vi "Lab Panel V4.83.vi"() -> ()   [LabVIEW 2013] (continued)
                n1629 = property on="O/I  LAB04-2" class="Bool (strict)"("DisabledEnum"=w2561) -> ()  [unwired: 2 in, 2 out]
                n1630 = property on="O/I  LAB03-2" class="Bool (strict)"("DisabledEnum"=w2563) -> ()  [unwired: 2 in, 2 out]
                n1631 = Not(x=w2568) -> (.not. x?=w2569:bool)
                n1632 = Not(x=w2567) -> (.not. x?=w2570:bool)
                n1633 = Not(x=w2566) -> (.not. x?=w2571:bool)
                n1634 = property on="RESULT LAB05-2" class="Bool (strict)"("Visible"=w2569) -> ()  [unwired: 2 in, 2 out]
                n1635 = property on="RESULT LAB05-1" class="Bool (strict)"("Visible"=w2570) -> ()  [unwired: 2 in, 2 out]
                n1636 = Not(x=w2565) -> (.not. x?=w2572:bool)
                n1637 = property on="RESULT LAB04-2" class="Bool (strict)"("Visible"=w2571) -> ()  [unwired: 2 in, 2 out]
                n1638 = Not(x=w2564) -> (.not. x?=w2573:bool)
                n1639 = property on="RESULT LAB04-1" class="Bool (strict)"("Visible"=w2572) -> ()  [unwired: 2 in, 2 out]
                n1640 = property on="RESULT LAB03-2" class="Bool (strict)"("Visible"=w2573) -> ()  [unwired: 2 in, 2 out]
              }
              frame #2 {
                # "disable calibrate if any test running"
                n1641 = Or(x=w2595, y=w2594) -> (x .or. y?=w2588:bool)
                n1642 = Or(x=w2597, y=w2596) -> (x .or. y?=w2590:bool)
                n1643 = Or(x=w2601, y=w2600) -> (x .or. y?=w2592:bool)
                n1644 = Or(x=w2599, y=w2598) -> (x .or. y?=w2591:bool)
                n1645 = Or(x=w2603, y=w2602) -> (x .or. y?=w2593:bool)
                n1646 = Or(x=w2591, y=w2590) -> (x .or. y?=w2589:bool)
                n1647 = Or(x=w2593, y=w2592) -> (x .or. y?=w2587:bool)
                n1648 = Or(x=w2589, y=w2588) -> (x .or. y?=w2586:bool)
                n1649 = Or(x=w2587, y=w2586) -> (x .or. y?=w2585:bool)
                n1650 = case shown="True" w2585 {
                  tunnel: [0 2] -> w2584
                  frame False {
                  }
                  frame True {
                  }
                }
                n1651 = property on="JIG TEST" class="Clust (strict)"("DisabledEnum"=w2584) -> ()  [unwired: 2 in, 2 out]
                n1652 = property on="Network Directory" class="Path"("DisabledEnum"=w2584) -> ()  [unwired: 2 in, 2 out]
                n1653 = property on="MAIL SETTINGS" class="Clust (strict)"("DisabledEnum"=w2584) -> ()  [unwired: 2 in, 2 out]
                n1654 = property on="CALIBRATE" class="Bool (strict)"("DisabledEnum"=w2584) -> ()  [unwired: 2 in, 2 out]
                n1655 = property on="ADMIN" class="Bool (strict)"("DisabledEnum"=w2584) -> ()  [unwired: 2 in, 2 out]
              }
            }
          }
          frame #8 {
            # "drive jigs"
            n1656 = stacked-sequence {
              frame #0 {
                # "jig on"
                n1657 = local read "jig cycle"() -> (w2611:dbl)
                n1658 = property on="JIG TEST" class="Clust (strict)"() -> ("DisabledEnum"=w2608:T14)  [unwired: 2 in, 2 out]
                n1659 = Equal?(x=w2608, y=2) -> (x = y?=w2607:bool)
                n1660 = Equal?(x=w2611, y=0) -> (x = y?=w2609:bool)
                n1661 = And(x=w2609, y=w2607) -> (x .and. y?=w2606:bool)
                n1662 = case shown="True" w2606 {
                  frame False {
                  }
                  frame True {
                    n1663 = local read "run lab01-1"() -> (w2622:bool)
                    n1664 = local read "run lab01-2"() -> (w2621:bool)
                    n1665 = local read "run lab02-1"() -> (w2620:bool)
                    n1666 = local read "run lab02-2"() -> (w2619:bool)
                    n1667 = local read "run lab03-1"() -> (w2618:bool)
                    n1668 = local read "run lab03-2"() -> (w2617:bool)
                    n1669 = local read "run lab04-1"() -> (w2616:bool)
                    n1670 = local read "run lab04-2"() -> (w2615:bool)
                    n1671 = local read "run lab05-1"() -> (w2614:bool)
                    n1672 = local read "run lab05-2"() -> (w2613:bool)
                    n1673 = local write "JIG LAB03-2"(w2617) -> ()
                    n1674 = local write "JIG LAB01-1"(w2622) -> ()
                    n1675 = local write "JIG LAB01-2"(w2621) -> ()
                    n1676 = local write "JIG LAB02-1"(w2620) -> ()
                    n1677 = local write "JIG LAB02-2"(w2619) -> ()
                    n1678 = local write "JIG LAB03-1"(w2618) -> ()
                    n1679 = local write "JIG LAB04-1"(w2616) -> ()
                    n1680 = local write "JIG LAB04-2"(w2615) -> ()
                    n1681 = local write "JIG LAB05-1"(w2614) -> ()
                    n1682 = local write "JIG LAB05-2"(w2613) -> ()
                  }
                }
              }
              frame #1 {
                # "jig off"
                n1683 = local read "jig cycle"() -> (w2629:dbl)
                n1684 = local read "on loops"() -> (w2628:dbl)
                n1685 = property on="JIG TEST" class="Clust (strict)"() -> ("DisabledEnum"=w2627:T14)  [unwired: 2 in, 2 out]
                n1686 = Equal?(x=w2627, y=2) -> (x = y?=w2625:bool)
                n1687 = Equal?(x=w2629, y=w2628) -> (x = y?=w2624:bool)
                n1688 = And(x=w2624, y=w2625) -> (x .and. y?=w2623:bool)
                n1689 = case shown="True" w2623 {
                  frame False {
                  }
                  frame True {
                    w2680 = FALSE
                    w2681 = TRUE
                    w2679 = 2
                    n1690 = local read "SELECT LAB05-2"() -> (w2670:T3)
                    n1691 = local read "SELECT LAB04-2"() -> (w2672:T3)
                    n1692 = local read "SELECT LAB04-1"() -> (w2673:T3)
                    n1693 = local read "SELECT LAB05-1"() -> (w2671:T3)
                    n1694 = local read "SELECT LAB03-2"() -> (w2674:T3)
                    n1695 = local read "SELECT LAB02-1"() -> (w2677:T3)
                    n1696 = local read "SELECT LAB03-1"() -> (w2675:T3)
                    n1697 = local read "SELECT LAB02-2"() -> (w2676:T3)
                    n1698 = local read "SELECT LAB01-2"() -> (w2678:T3)
                    n1699 = local read "run lab05-1"() -> (w2640:bool)
                    n1700 = local read "run lab05-2"() -> (w2639:bool)
                    n1701 = local read "SELECT LAB01-1"() -> (w2682:T3)
                    n1702 = local read "run lab04-2"() -> (w2641:bool)
                    n1703 = local read "run lab04-1"() -> (w2642:bool)
                    n1704 = local read "run lab01-1"() -> (w2658:bool)
                    n1705 = local read "run lab01-2"() -> (w2647:bool)
                    n1706 = local read "run lab03-2"() -> (w2643:bool)
                    n1707 = local read "run lab03-1"() -> (w2644:bool)
                    n1708 = local read "run lab02-1"() -> (w2646:bool)
                    n1709 = local read "run lab02-2"() -> (w2645:bool)
                    n1710 = Equal?(x=w2679, y=w2675) -> (x = y?=w2653:bool)
                    n1711 = Equal?(x=w2679, y=w2674) -> (x = y?=w2652:bool)
                    n1712 = Equal?(x=w2679, y=w2673) -> (x = y?=w2651:bool)
                    n1713 = Equal?(x=w2679, y=w2672) -> (x = y?=w2650:bool)
                    n1714 = Equal?(x=w2679, y=w2671) -> (x = y?=w2649:bool)
                    n1715 = Equal?(x=w2679, y=w2670) -> (x = y?=w2648:bool)
                    n1716 = Equal?(x=w2679, y=w2682) -> (x = y?=w2659:bool)
                    n1717 = Equal?(x=w2679, y=w2677) -> (x = y?=w2655:bool)
                    n1718 = Equal?(x=w2679, y=w2676) -> (x = y?=w2654:bool)
                    n1719 = Equal?(x=w2679, y=w2678) -> (x = y?=w2656:bool)
                    n1720 = And(x=w2650, y=w2641) -> (x .and. y?=w2632:bool)
                    n1721 = And(x=w2653, y=w2644) -> (x .and. y?=w2635:bool)
                    n1722 = And(x=w2651, y=w2642) -> (x .and. y?=w2633:bool)
                    n1723 = And(x=w2648, y=w2639) -> (x .and. y?=w2630:bool)
                    n1724 = And(x=w2654, y=w2645) -> (x .and. y?=w2636:bool)
                    n1725 = And(x=w2652, y=w2643) -> (x .and. y?=w2634:bool)
                    n1726 = And(x=w2649, y=w2640) -> (x .and. y?=w2631:bool)
                    n1727 = And(x=w2656, y=w2647) -> (x .and. y?=w2638:bool)
                    n1728 = And(x=w2659, y=w2658) -> (x .and. y?=w2657:bool)
                    n1729 = And(x=w2655, y=w2646) -> (x .and. y?=w2637:bool)
                    n1730 = Select(t=w2681, s=w2657, f=w2680) -> (s? t:f=w2660:bool)
                    n1731 = Select(t=w2681, s=w2638, f=w2680) -> (s? t:f=w2661:bool)
                    n1732 = Select(t=w2681, s=w2637, f=w2680) -> (s? t:f=w2662:bool)
                    n1733 = Select(t=w2681, s=w2636, f=w2680) -> (s? t:f=w2663:bool)
                    n1734 = Select(t=w2681, s=w2635, f=w2680) -> (s? t:f=w2664:bool)
                    n1735 = Select(t=w2681, s=w2634, f=w2680) -> (s? t:f=w2665:bool)
                    n1736 = Select(t=w2681, s=w2633, f=w2680) -> (s? t:f=w2666:bool)
                    n1737 = Select(t=w2681, s=w2632, f=w2680) -> (s? t:f=w2667:bool)
                    n1738 = Select(t=w2681, s=w2631, f=w2680) -> (s? t:f=w2668:bool)
                    n1739 = Select(t=w2681, s=w2630, f=w2680) -> (s? t:f=w2669:bool)
                    n1740 = local write "JIG LAB03-2"(w2665) -> ()
                    n1741 = local write "JIG LAB02-1"(w2662) -> ()
                    n1742 = local write "JIG LAB02-2"(w2663) -> ()
                    n1743 = local write "JIG LAB01-2"(w2661) -> ()
                    n1744 = local write "JIG LAB03-1"(w2664) -> ()
                    n1745 = local write "JIG LAB01-1"(w2660) -> ()
                    n1746 = local write "JIG LAB05-2"(w2669) -> ()
                    n1747 = local write "JIG LAB04-1"(w2666) -> ()
                    n1748 = local write "JIG LAB05-1"(w2668) -> ()
                    n1749 = local write "JIG LAB04-2"(w2667) -> ()
                  }
                }
              }
            }
          }
          frame #9 {
            # "enable  jig test output if no test busy"
            n1750 = property on="JIG TEST" class="Clust (strict)"() -> ("DisabledEnum"=w2685:T14)  [unwired: 2 in, 2 out]
            n1751 = Equal?(x=w2685, y=0) -> (x = y?=w2683:bool)
            n1752 = case shown="True" w2683 {
              frame False {
              }
              frame True {
                n1753 = local read "JIG TEST"() -> (w2696:T11)
                n1754 = Unbundle(w2696) -> ("LAB01-1"=w2695:bool, "LAB01-2"=w2694:bool, "LAB02-1"=w2693:bool, "LAB02-2"=w2692:bool, "LAB03-1"=w2691:bool, "LAB03-2"=w2690:bool, "LAB04-1"=w2689:bool, "LAB04-2"=w2688:bool, "LAB05-1"=w2687:bool, "LAB05-2"=w2686:bool)
                n1755 = local write "JIG LAB05-1"(w2687) -> ()
                n1756 = local write "JIG LAB05-2"(w2686) -> ()
                n1757 = local write "JIG LAB04-1"(w2689) -> ()
                n1758 = local write "JIG LAB04-2"(w2688) -> ()
                n1759 = local write "JIG LAB03-2"(w2690) -> ()
                n1760 = local write "JIG LAB01-1"(w2695) -> ()
                n1761 = local write "JIG LAB02-1"(w2693) -> ()
                n1762 = local write "JIG LAB03-1"(w2691) -> ()
                n1763 = local write "JIG LAB01-2"(w2694) -> ()
                n1764 = local write "JIG LAB02-2"(w2692) -> ()
              }
            }
          }
          frame #10 {
            # "drive digital output"
            n1765 = local read "O/I  LAB05-2"() -> (w2703:bool)
            n1766 = local read "O/I  LAB05-1"() -> (w2705:bool)
            n1767 = local read "JIG LAB05-2"() -> (w2702:bool)
            n1768 = local read "O/I  LAB04-2"() -> (w2707:bool)
            n1769 = local read "JIG LAB05-1"() -> (w2704:bool)
            n1770 = local read "JIG LAB04-2"() -> (w2706:bool)
            n1771 = local read "O/I  LAB03-1"() -> (w2712:bool)
            n1772 = local read "O/I  LAB04-1"() -> (w2708:bool)
            n1773 = local read "O/I  LAB02-1"() -> (w2716:bool)
            n1774 = local read "O/I  LAB02-2"() -> (w2714:bool)
            n1775 = local read "O/I  LAB03-2"() -> (w2710:bool)
            n1776 = local read "JIG LAB04-1"() -> (w2701:bool)
            n1777 = local read "JIG LAB03-2"() -> (w2709:bool)
            n1778 = local read "O/I  LAB01-2"() -> (w2718:bool)
            n1779 = local read "JIG LAB02-1"() -> (w2715:bool)
            n1780 = local read "JIG LAB02-2"() -> (w2713:bool)
            n1781 = local read "JIG LAB03-1"() -> (w2711:bool)
            n1782 = local read "O/I  LAB01-1"() -> (w2720:bool)
            n1783 = local read "JIG LAB01-2"() -> (w2717:bool)
            n1784 = local read "JIG LAB01-1"() -> (w2719:bool)
            n1785 = Build Array(w2707, w2706, w2705, w2704, w2703, w2702) -> (w2698:bool[])
            n1786 = Build Array(w2713, w2712, w2711, w2710, w2709, w2708, w2701) -> (w2699:bool[])
            n1787 = Build Array(w2720, w2719, w2718, w2717, w2716, w2715, w2714) -> (w2700:bool[])
            n1788 = local read "simulate"() -> (w2697:bool)
            n1789 = case shown="False" w2697 {
              tunnel: w2700 -> [w2723 _]
              tunnel: w2699 -> [w2722 _]
              tunnel: w2698 -> [w2721 _]
              frame False {
                n1790 = call "sub vi - Drive Relays All v6.vi"("Array #2"=w2721, "Array #1"=w2722, "Array #0"=w2723) -> ()  [unwired: 8 in, 1 out]
              }
              frame True {
              }
            }
          }
          frame #11 {
            # "get analog values"
            n1791 = local read "on loops"() -> (w2730:dbl)
            n1792 = local read "jig cycle"() -> (w2727:dbl)
            n1793 = Add(x=w2730, y=1) -> (x+y=w2728:dbl)
            n1794 = Equal?(x=w2727, y=1) -> (x = y?=w2725:bool)
            n1795 = Equal?(x=w2727, y=w2728) -> (x = y?=w2726:bool)
            n1796 = Or(x=w2725, y=w2726) -> (x .or. y?=w2724:bool)
            n1797 = case shown="True" w2724 {
              frame False {
              }
              frame True {
                n1798 = local read "simulate"() -> (w2734:bool)
                n1799 = case shown="False" w2734 {
                  tunnel: [w2750 errorcluster[] [] ("array ERROR")] -> w2742
                  tunnel: [w2749 0.3 ("Analog loop time")] -> w2741
                  tunnel: [w2748 dynamicdata[] [] ("array GRAPH")] -> w2740
                  tunnel: [w2747 w2752] -> w2739
                  tunnel: [w2746 w2752] -> w2738
                  tunnel: [w2745 w2752] -> w2737
                  tunnel: [w2744 w2752] -> w2736
                  tunnel: [w2743 w2752] -> w2735
                  frame False {
                    n1800 = call "sub vi - Read Analog All v8.vi"() -> ("Analog loop time"=w2749:dbl, "array GRAPH"=w2748:dynamicdata[], "LAB01"=w2747:T23, "LAB02"=w2746:T24, "LAB03"=w2745:T25, "LAB04"=w2744:T26, "array ERROR"=w2750:errorcluster[], "LAB05"=w2743:T27)  [unwired: 8 in]
                  }
                  frame True {
                    w2752 = T27 {"LAB05-1 (A)"=10.0, "LAB05-1 (V)"=220.0, "LAB05-1 (PF)"=0.5, "LAB05-2 (A)"=15.0, "LAB05-2 (V)"=225.0, "LAB05-2 (PF)"=0.6} ("LAB05")
                  }
                }
                n1801 = local read "simulate"() -> (w2733:bool)
                n1802 = stacked-sequence {
                  tunnel: w2742 -> [w2759 _ _ _ _ _]
                  tunnel: w2741 -> [w2758 _ _ _ _ _]
                  tunnel: w2740 -> [w2757 _ _ _ _ _]
                  tunnel: w2739 -> [_ w2806 _ _ _ _]
                  tunnel: w2738 -> [_ _ w2813 _ _ _]
                  tunnel: w2737 -> [_ _ _ w2842 _ _]
                  tunnel: w2736 -> [_ _ _ _ w2869 _]
                  tunnel: w2735 -> [_ _ _ _ _ w2898]
                  tunnel: w2733 -> [_ w2784 w2812 w2840 w2868 w2896]
                  tunnel: T9 {"1  (A) cal"=1.0, "1 (V) cal"=1.0, "1 (PF) cal"=1.0, "1 (TL) cal"=1.0, "1 (TN) cal"=1.0, "2 (A) cal"=1.0, "2 (V) cal"=1.0, "2 (PF) cal"=1.0, "2 (TL) cal"=1.0, "2 (TN) cal"=1.0} ("CAL LAB01") -> [_ w2783 w2811 w2839 w2867 w2895]
                  frame #0 {
                    n1803 = local write "AI"(TRUE) -> ()
                    n1804 = global write "Global 1.vi" "RATE(Hz)"("RATE (Hz)") -> ()
                    n1805 = global write "Global 1.vi" "SAMPLES"("SAMPLES") -> ()
                    n1806 = Index Array(array=w2757, index=6) -> (element=→"LAB04-1 (GRAPH)":dynamicdata)
                    n1807 = Index Array(array=w2757, index=7) -> (element=→"LAB04-2 (GRAPH)":dynamicdata)
                    n1808 = Index Array(array=w2757, index=9) -> (element=→"LAB05-2 (GRAPH)":dynamicdata)
                    n1809 = Index Array(array=w2757, index=8) -> (element=→"LAB05-1 (GRAPH)":dynamicdata)
                    n1810 = Index Array(array=w2757, index=5) -> (element=→"LAB03-2 (GRAPH)":dynamicdata)
                    n1811 = Index Array(array=w2757, index=0) -> (element=→"LAB01-1 (GRAPH)":dynamicdata)
                    n1812 = Index Array(array=w2757, index=1) -> (element=→"LAB01-2 (GRAPH)":dynamicdata)
                    n1813 = Index Array(array=w2757, index=2) -> (element=→"LAB02-1 (GRAPH)":dynamicdata)
                    n1814 = Index Array(array=w2757, index=3) -> (element=→"LAB02-2 (GRAPH)":dynamicdata)
                    n1815 = Index Array(array=w2757, index=4) -> (element=→"LAB03-1 (GRAPH)":dynamicdata)
                    "AI loop time" <- w2758
                    "Analog Error Array" <- w2759
                  }
                  frame #1 {
                    n1816 = Unbundle By Name(w2806) -> ("LAB05-1 (A)"=w2804:dbl, "LAB05-1 (V)"=w2803:dbl, "LAB05-1 (PF)"=w2802:dbl, "LAB05-2 (A)"=w2801:dbl, "LAB05-2 (V)"=w2800:dbl, "LAB05-2 (PF)"=w2799:dbl)
                    n1817 = case shown="False" w2784 {
                      tunnel: [w2807 w2808] -> w2805
                      tunnel: w2783 -> [_ w2808]
                      frame False {
                        n1818 = local read "CAL LAB01"() -> (w2807:T9)
                      }
                      frame True {
                      }
                    }
                    n1819 = Unbundle By Name(w2805) -> ("1  (A) cal"=w2798:dbl, "1 (V) cal"=w2797:dbl, "1 (PF) cal"=w2796:dbl, "2 (A) cal"=w2795:dbl, "2 (V) cal"=w2794:dbl, "2 (PF) cal"=w2793:dbl)  [unwired: 4 out]
                    n1820 = Multiply(x=w2804, y=w2798) -> (x*y=w2791:dbl)
                    n1821 = Multiply(x=w2803, y=w2797) -> (x*y=w2790:dbl)
                    n1822 = Multiply(x=w2802, y=w2796) -> (x*y=w2789:dbl)
                    n1823 = Multiply(x=w2801, y=w2795) -> (x*y=w2787:dbl)
                    n1824 = Multiply(x=w2800, y=w2794) -> (x*y=w2786:dbl)
                    n1825 = Multiply(x=w2799, y=w2793) -> (x*y=w2785:dbl)
                    n1826 = local read "SIG LAB01-1"() -> (w2792:T2)
                    n1827 = local read "SIG LAB01-2"() -> (w2788:T2)
                    n1828 = Bundle By Name(cluster=w2792, "AMPS"=w2791, "VOLTS"=w2790, "PF"=w2789) -> (w2782:T2)
                    n1829 = Bundle By Name(cluster=w2788, "AMPS"=w2787, "VOLTS"=w2786, "PF"=w2785) -> (w2781:T2)
                    n1830 = global write "Global display 1.vi" "SIG LAB01-2"(w2781) -> ()
                    n1831 = global write "Global display 1.vi" "SIG LAB01-1"(w2782) -> ()
                    n1832 = local write "SIG LAB01-2"(w2781) -> ()
                    n1833 = local write "SIG LAB01-1"(w2782) -> ()
                  }
                  frame #2 {
                    n1834 = Unbundle By Name(w2813) -> ("LAB05-1 (A)"=w2833:dbl, "LAB05-1 (V)"=w2832:dbl, "LAB05-1 (PF)"=w2831:dbl, "LAB05-2 (A)"=w2830:dbl, "LAB05-2 (V)"=w2829:dbl, "LAB05-2 (PF)"=w2828:dbl)
                    n1835 = case shown="True" w2812 {
                      tunnel: [w2835 w2836] -> w2834
                      tunnel: w2811 -> [_ w2836]
                      frame False {
                        n1836 = local read "CAL LAB02"() -> (w2835:T10)
                      }
                      frame True {
                      }
                    }
                    n1837 = Unbundle By Name(w2834) -> ("1  (A) cal"=w2827:dbl, "1 (V) cal"=w2826:dbl, "1 (PF) cal"=w2825:dbl, "2 (A) cal"=w2824:dbl, "2 (V) cal"=w2823:dbl, "2 (PF) cal"=w2822:dbl)  [unwired: 4 out]
                    n1838 = Multiply(x=w2833, y=w2827) -> (x*y=w2820:dbl)
                    n1839 = Multiply(x=w2832, y=w2826) -> (x*y=w2819:dbl)
                    n1840 = Multiply(x=w2831, y=w2825) -> (x*y=w2818:dbl)
                    n1841 = Multiply(x=w2830, y=w2824) -> (x*y=w2816:dbl)
                    n1842 = Multiply(x=w2829, y=w2823) -> (x*y=w2815:dbl)
                    n1843 = Multiply(x=w2828, y=w2822) -> (x*y=w2814:dbl)
                    n1844 = local read "SIG LAB02-1"() -> (w2821:T2)
                    n1845 = local read "SIG LAB02-2"() -> (w2817:T2)
                    n1846 = Bundle By Name(cluster=w2821, "AMPS"=w2820, "VOLTS"=w2819, "PF"=w2818) -> (w2810:T2)
                    n1847 = Bundle By Name(cluster=w2817, "AMPS"=w2816, "VOLTS"=w2815, "PF"=w2814) -> (w2809:T2)
                    n1848 = global write "Global display 1.vi" "SIG LAB02-1"(w2810) -> ()
                    n1849 = local write "SIG LAB02-2"(w2809) -> ()
                    n1850 = global write "Global display 1.vi" "SIG LAB02-2"(w2809) -> ()
                    n1851 = local write "SIG LAB02-1"(w2810) -> ()
                  }
                  frame #3 {
                    n1852 = Unbundle By Name(w2842) -> ("LAB05-1 (A)"=w2861:dbl, "LAB05-1 (V)"=w2860:dbl, "LAB05-1 (PF)"=w2859:dbl, "LAB05-2 (A)"=w2858:dbl, "LAB05-2 (V)"=w2857:dbl, "LAB05-2 (PF)"=w2856:dbl)
                    n1853 = case shown="True" w2840 {
                      tunnel: [w2863 w2864] -> w2862
                      tunnel: w2839 -> [_ w2864]
                      frame False {
                        n1854 = local read "CAL LAB03"() -> (w2863:T9)
                      }
                      frame True {
                      }
                    }
                    n1855 = Unbundle By Name(w2862) -> ("1  (A) cal"=w2855:dbl, "1 (V) cal"=w2854:dbl, "1 (PF) cal"=w2853:dbl, "2 (A) cal"=w2852:dbl, "2 (V) cal"=w2851:dbl, "2 (PF) cal"=w2850:dbl)  [unwired: 4 out]
                    n1856 = Multiply(x=w2861, y=w2855) -> (x*y=w2848:dbl)
                    n1857 = Multiply(x=w2860, y=w2854) -> (x*y=w2841:dbl)
                    n1858 = Multiply(x=w2859, y=w2853) -> (x*y=w2847:dbl)
                    n1859 = Multiply(x=w2858, y=w2852) -> (x*y=w2845:dbl)
                    n1860 = Multiply(x=w2857, y=w2851) -> (x*y=w2844:dbl)
                    n1861 = Multiply(x=w2856, y=w2850) -> (x*y=w2843:dbl)
                    n1862 = local read "SIG LAB03-1"() -> (w2849:T2)
                    n1863 = local read "SIG LAB03-2"() -> (w2846:T2)
                    n1864 = Bundle By Name(cluster=w2849, "AMPS"=w2848, "VOLTS"=w2841, "PF"=w2847) -> (w2838:T2)
                    n1865 = Bundle By Name(cluster=w2846, "AMPS"=w2845, "VOLTS"=w2844, "PF"=w2843) -> (w2837:T2)
                    n1866 = global write "Global display 1.vi" "SIG LAB03-1"(w2838) -> ()
                    n1867 = global write "Global display 1.vi" "SIG LAB03-2"(w2837) -> ()
                    n1868 = local write "SIG LAB03-2"(w2837) -> ()
                    n1869 = local write "SIG LAB03-1"(w2838) -> ()
                  }
                  frame #4 {
                    n1870 = Unbundle By Name(w2869) -> ("LAB05-1 (A)"=w2889:dbl, "LAB05-1 (V)"=w2888:dbl, "LAB05-1 (PF)"=w2887:dbl, "LAB05-2 (A)"=w2886:dbl, "LAB05-2 (V)"=w2885:dbl, "LAB05-2 (PF)"=w2884:dbl)
                    n1871 = case shown="False" w2868 {
                      tunnel: [w2891 w2892] -> w2890
                      tunnel: w2867 -> [_ w2892]
                      frame False {
                        n1872 = local read "CAL LAB04"() -> (w2891:T9)
                      }
                      frame True {
                      }
                    }
                    n1873 = Unbundle By Name(w2890) -> ("1  (A) cal"=w2883:dbl, "1 (V) cal"=w2882:dbl, "1 (PF) cal"=w2881:dbl, "2 (A) cal"=w2880:dbl, "2 (V) cal"=w2879:dbl, "2 (PF) cal"=w2878:dbl)  [unwired: 4 out]
                    n1874 = Multiply(x=w2889, y=w2883) -> (x*y=w2876:dbl)
                    n1875 = Multiply(x=w2888, y=w2882) -> (x*y=w2875:dbl)
                    n1876 = Multiply(x=w2887, y=w2881) -> (x*y=w2874:dbl)
                    n1877 = Multiply(x=w2886, y=w2880) -> (x*y=w2872:dbl)
                    n1878 = Multiply(x=w2885, y=w2879) -> (x*y=w2871:dbl)
                    n1879 = Multiply(x=w2884, y=w2878) -> (x*y=w2870:dbl)
                    n1880 = local read "SIG LAB04-1"() -> (w2877:T2)
                    n1881 = local read "SIG LAB04-2"() -> (w2873:T2)
                    n1882 = Bundle By Name(cluster=w2877, "AMPS"=w2876, "VOLTS"=w2875, "PF"=w2874) -> (w2866:T2)
                    n1883 = Bundle By Name(cluster=w2873, "AMPS"=w2872, "VOLTS"=w2871, "PF"=w2870) -> (w2865:T2)
                    n1884 = global write "Global display 1.vi" "SIG LAB04-2"(w2865) -> ()
                    n1885 = global write "Global display 1.vi" "SIG LAB04-1"(w2866) -> ()
                    n1886 = local write "SIG LAB04-2"(w2865) -> ()
                    n1887 = local write "SIG LAB04-1"(w2866) -> ()
                  }
                  frame #5 {
                    n1888 = Unbundle By Name(w2898) -> ("LAB05-1 (A)"=w2917:dbl, "LAB05-1 (V)"=w2897:dbl, "LAB05-1 (PF)"=w2916:dbl, "LAB05-2 (A)"=w2915:dbl, "LAB05-2 (V)"=w2914:dbl, "LAB05-2 (PF)"=w2913:dbl)
                    n1889 = case shown="False" w2896 {
                      tunnel: [w2919 w2920] -> w2918
                      tunnel: w2895 -> [_ w2920]
                      frame False {
                        n1890 = local read "CAL LAB05"() -> (w2919:T9)
                      }
                      frame True {
                      }
                    }
                    n1891 = Unbundle By Name(w2918) -> ("1  (A) cal"=w2912:dbl, "1 (V) cal"=w2911:dbl, "1 (PF) cal"=w2910:dbl, "2 (A) cal"=w2909:dbl, "2 (V) cal"=w2908:dbl, "2 (PF) cal"=w2907:dbl)  [unwired: 4 out]
                    n1892 = Multiply(x=w2917, y=w2912) -> (x*y=w2905:dbl)
                    n1893 = Multiply(x=w2897, y=w2911) -> (x*y=w2904:dbl)
                    n1894 = Multiply(x=w2916, y=w2910) -> (x*y=w2903:dbl)
                    n1895 = Multiply(x=w2915, y=w2909) -> (x*y=w2901:dbl)
                    n1896 = Multiply(x=w2914, y=w2908) -> (x*y=w2900:dbl)
                    n1897 = Multiply(x=w2913, y=w2907) -> (x*y=w2899:dbl)
                    n1898 = local read "SIG LAB05-1"() -> (w2906:T2)
                    n1899 = local read "SIG LAB05-2"() -> (w2902:T2)
                    n1900 = Bundle By Name(cluster=w2906, "AMPS"=w2905, "VOLTS"=w2904, "PF"=w2903) -> (w2894:T2)
                    n1901 = Bundle By Name(cluster=w2902, "AMPS"=w2901, "VOLTS"=w2900, "PF"=w2899) -> (w2893:T2)
                    n1902 = global write "Global display 1.vi" "SIG LAB05-1"(w2894) -> ()
                    n1903 = global write "Global display 1.vi" "SIG LAB05-2"(w2893) -> ()
                    n1904 = local write "SIG LAB05-2"(w2893) -> ()
                    n1905 = local write "SIG LAB05-1"(w2894) -> ()
                  }
                }
              }
            }
          }
          frame #12 {
            # "save test data to file"
            n1906 = Get Date/Time In Seconds() -> (seconds since 1Jan1904=w2921:timestamp)
            "File Time Stamp" <- w2921
            n1907 = local read "on loops"() -> (w2940:dbl)
            n1908 = local read "jig cycle"() -> (w2937:dbl)
            n1909 = Format Date/Time String(time format string (%c)="%H:%M%:%S", seconds (now)=w2921) -> (date/time string=w2925:string)  [unwired: 1 in]
            n1910 = Add(x=w2940, y=2) -> (x+y=w2938:dbl)
            n1911 = Build Array(w2925) -> (w2924:string[])
            n1912 = Equal?(x=w2937, y=1) -> (x = y?=w2923:bool)
            n1913 = Equal?(x=w2937, y=w2938) -> (x = y?=w2922:bool)
            n1914 = stacked-sequence {
              tunnel: w2936 -> [w2946 _ _ _ _ _ _ _ _ _]
              tunnel: w2935 -> [_ w3022 _ _ _ _ _ _ _ _]
              tunnel: w2934 -> [_ _ w3102 _ _ _ _ _ _ _]
              tunnel: w2933 -> [_ _ _ w3182 _ _ _ _ _ _]
              tunnel: w2932 -> [_ _ _ _ w3262 _ _ _ _ _]
              tunnel: w2931 -> [_ _ _ _ _ w3342 _ _ _ _]
              tunnel: w2930 -> [_ _ _ _ _ _ w3422 _ _ _]
              tunnel: w2929 -> [_ _ _ _ _ _ _ w3502 _ _]
              tunnel: w2928 -> [_ _ _ _ _ _ _ _ w3582 _]
              tunnel: w2927 -> [_ _ _ _ _ _ _ _ _ w3662]
              tunnel: w2924 -> [w2945 w3026 w3106 w3186 w3266 w3346 w3426 w3506 w3586 w3666]
              tunnel: w2923 -> [w2944 w3025 w3105 w3185 w3265 w3345 w3425 w3505 w3585 w3665]
              tunnel: w2922 -> [w2943 w3024 w3104 w3184 w3264 w3344 w3424 w3504 w3584 w3664]
              tunnel: w2921 -> [w2942 w3023 w3103 w3183 w3263 w3343 w3423 w3503 w3583 w3663]
              frame #0 {
                n1915 = case shown="True" w2946 {
                  tunnel: w2945 -> [_ w2951]
                  tunnel: w2944 -> [_ w2950]
                  tunnel: w2943 -> [_ w2948]
                  tunnel: w2942 -> [_ w2947]
                  frame False {
                  }
                  frame True {
                    n1916 = local read "DISP LAB01-1"() -> (w2952:T4)
                    n1917 = local read "SIG LAB01-1"() -> (w2953:T2)
                    n1918 = local read "ON L01-1"() -> (w2949:cluster{"amps":dbl, "volts":dbl, "pf":dbl})
                    n1919 = Unbundle(w2953) -> ("AMPS"=w2959:dbl, "VOLTS"=w2957:dbl, "PF"=w2956:dbl, "Tmp Live"=w2955:dbl, "Tmp Neut"=w2958:dbl)
                    n1920 = Unbundle(w2952) -> ("CYCLE"=w2954:dbl)  [unwired: 2 out]
                    n1921 = stacked-sequence {
                      tunnel: w2959 -> [w2963 w2982]
                      tunnel: w2958 -> [_ w2981]
                      tunnel: w2957 -> [w2962 w2980]
                      tunnel: w2956 -> [w2961 w2979]
                      tunnel: w2955 -> [_ w2978]
                      tunnel: w2954 -> [_ w2977]
                      tunnel: w2951 -> [_ w2976]
                      tunnel: w2950 -> [w2964 _]
                      tunnel: w2949 -> [w2960 w2974]
                      tunnel: w2948 -> [_ w2975]
                      tunnel: w2947 -> [_ w2970]
                      frame #0 {
                        n1922 = case shown="True" w2964 {
                          tunnel: w2963 -> [_ w2969]
                          tunnel: w2962 -> [_ w2968]
                          tunnel: w2961 -> [_ w2967]
                          tunnel: w2960 -> [_ w2965]
                          frame False {
                          }
                          frame True {
                            n1923 = Bundle(cluster=w2965, "amps"=w2969, "volts"=w2968, "pf"=w2967) -> (w2966:cluster{"amps":dbl, "volts":dbl, "pf":dbl})
                            n1924 = local write "ON L01-1"(w2966) -> ()
                          }
                        }
                      }
                      frame #1 {
                        n1925 = Unbundle(w2974) -> ("amps"=w2973:dbl, "volts"=w2972:dbl, "pf"=w2971:dbl)
                        n1926 = case shown="True" w2975 {
                          tunnel: w2982 -> [_ w2983]
                          tunnel: w2981 -> [_ w3021]
                          tunnel: w2980 -> [_ _]
                          tunnel: w2979 -> [_ _]
                          tunnel: w2978 -> [_ w3020]
                          tunnel: w2977 -> [_ w3019]
                          tunnel: w2976 -> [_ w2987]
                          tunnel: w2973 -> [_ w2984]
                          tunnel: w2972 -> [_ w3016]
                          tunnel: w2971 -> [_ w3015]
                          tunnel: w2970 -> [_ w2985]
                          frame False {
                          }
                          frame True {
                            n1927 = local read "TDMS LAB01-1"() -> (w3018:refnum<k34>)
                            n1928 = Build Array(w3016) -> (w3012:dbl[])
                            n1929 = Build Array(w3015) -> (w3011:dbl[])
                            n1930 = Build Array(w3020) -> (w3010:dbl[])
                            n1931 = Build Array(w3021) -> (w3009:dbl[])
                            n1932 = Build Array(w2984) -> (w3014:dbl[])
                            n1933 = Build Array(w2983) -> (w3013:dbl[])
                            n1934 = Build Array(w3019) -> (w3008:dbl[])
                            n1935 = Build Array("AMPS ON", "AMPS OFF", "VOLTS", "PF", "TEMP Live", "TEMP Neut", "CYCLE") -> (w2992:string[])
                            n1936 = Bundle By Name("Y"=w3014, "t0"=w2985) -> (w3007:waveform(dbl))  [unwired: 1 in]
                            n1937 = Bundle By Name("Y"=w3013, "t0"=w2985) -> (w3006:waveform(dbl))  [unwired: 1 in]
                            n1938 = Bundle By Name("Y"=w3012, "t0"=w2985) -> (w3005:waveform(dbl))  [unwired: 1 in]
                            n1939 = Bundle By Name("Y"=w3011, "t0"=w2985) -> (w3004:waveform(dbl))  [unwired: 1 in]
                            n1940 = Bundle By Name("Y"=w3010, "t0"=w2985) -> (w3003:waveform(dbl))  [unwired: 1 in]
                            n1941 = Bundle By Name("Y"=w3009, "t0"=w2985) -> (w3002:waveform(dbl))  [unwired: 1 in]
                            n1942 = Bundle By Name("Y"=w3008, "t0"=w2985) -> (w3001:waveform(dbl))  [unwired: 1 in]
                            n1943 = Build Array(w3007, w3006, w3005, w3004, w3003, w3002, w3001) -> (w3000:waveform(dbl)[])
                            n1944 = TDMS Write(0:w3018, 5:"TEST VALUES", 7:w2992, 9:w3000) -> (4:w2991:refnum<k34>, 6:w2990:string, 15:w2989:errorcluster)  [unwired: 2 in, 1 out]
                            n1945 = TDMS Write(0:w2991, 5:w2990, 7:"TIME", 9:w2987, 11:w2989) -> (15:w2986:errorcluster)  [unwired: 1 in, 3 out]
                            n1946 = local write "data file error"(w2986) -> ()
                          }
                        }
                      }
                    }
                  }
                }
              }
              frame #1 {
                n1947 = case shown="True" w3022 {
                  tunnel: w3026 -> [_ w3031]
                  tunnel: w3025 -> [_ w3030]
                  tunnel: w3024 -> [_ w3028]
                  tunnel: w3023 -> [_ w3027]
                  frame False {
                  }
                  frame True {
                    n1948 = local read "DISP LAB01-2"() -> (w3032:T4)
                    n1949 = local read "SIG LAB01-2"() -> (w3033:T2)
                    n1950 = local read "ON L01-2"() -> (w3029:cluster{"amps":dbl, "volts":dbl, "pf":dbl})
                    n1951 = Unbundle(w3033) -> ("AMPS"=w3039:dbl, "VOLTS"=w3037:dbl, "PF"=w3036:dbl, "Tmp Live"=w3035:dbl, "Tmp Neut"=w3038:dbl)
                    n1952 = Unbundle(w3032) -> ("CYCLE"=w3034:dbl)  [unwired: 2 out]
                    n1953 = stacked-sequence {
                      tunnel: w3039 -> [w3043 w3062]
                      tunnel: w3038 -> [_ w3061]
                      tunnel: w3037 -> [w3042 w3060]
                      tunnel: w3036 -> [w3041 w3059]
                      tunnel: w3035 -> [_ w3058]
                      tunnel: w3034 -> [_ w3057]
                      tunnel: w3031 -> [_ w3056]
                      tunnel: w3030 -> [w3044 _]
                      tunnel: w3029 -> [w3040 w3054]
                      tunnel: w3028 -> [_ w3055]
                      tunnel: w3027 -> [_ w3050]
                      frame #0 {
                        n1954 = case shown="True" w3044 {
                          tunnel: w3043 -> [_ w3049]
                          tunnel: w3042 -> [_ w3048]
                          tunnel: w3041 -> [_ w3047]
                          tunnel: w3040 -> [_ w3045]
                          frame False {
                          }
                          frame True {
                            n1955 = Bundle(cluster=w3045, "amps"=w3049, "volts"=w3048, "pf"=w3047) -> (w3046:cluster{"amps":dbl, "volts":dbl, "pf":dbl})
                            n1956 = local write "ON L01-2"(w3046) -> ()
                          }
                        }
                      }
                      frame #1 {
                        n1957 = Unbundle(w3054) -> ("amps"=w3053:dbl, "volts"=w3052:dbl, "pf"=w3051:dbl)
                        n1958 = case shown="True" w3055 {
                          tunnel: w3062 -> [_ w3094]
                          tunnel: w3061 -> [_ w3101]
                          tunnel: w3060 -> [_ _]
                          tunnel: w3059 -> [_ _]
                          tunnel: w3058 -> [_ w3100]
                          tunnel: w3057 -> [_ w3099]
                          tunnel: w3056 -> [_ w3064]
                          tunnel: w3053 -> [_ w3096]
                          tunnel: w3052 -> [_ w3095]
                          tunnel: w3051 -> [_ w3093]
                          tunnel: w3050 -> [_ w3085]
                          frame False {
                          }
                          frame True {
                            n1959 = local read "TDMS LAB01-2"() -> (w3098:refnum<k34>)
                            n1960 = Build Array(w3095) -> (w3090:dbl[])
                            n1961 = Build Array(w3093) -> (w3089:dbl[])
                            n1962 = Build Array(w3100) -> (w3088:dbl[])
                            n1963 = Build Array(w3101) -> (w3087:dbl[])
                            n1964 = Build Array(w3096) -> (w3092:dbl[])
                            n1965 = Build Array(w3094) -> (w3091:dbl[])
                            n1966 = Build Array(w3099) -> (w3086:dbl[])
                            n1967 = Build Array("AMPS ON", "AMPS OFF", "VOLTS", "PF", "TEMP Live", "TEMP Neut", "CYCLE") -> (w3069:string[])
                            n1968 = Bundle By Name("Y"=w3092, "t0"=w3085) -> (w3084:waveform(dbl))  [unwired: 1 in]
                            n1969 = Bundle By Name("Y"=w3091, "t0"=w3085) -> (w3083:waveform(dbl))  [unwired: 1 in]
                            n1970 = Bundle By Name("Y"=w3090, "t0"=w3085) -> (w3082:waveform(dbl))  [unwired: 1 in]
                            n1971 = Bundle By Name("Y"=w3089, "t0"=w3085) -> (w3081:waveform(dbl))  [unwired: 1 in]
                            n1972 = Bundle By Name("Y"=w3088, "t0"=w3085) -> (w3080:waveform(dbl))  [unwired: 1 in]
                            n1973 = Bundle By Name("Y"=w3087, "t0"=w3085) -> (w3079:waveform(dbl))  [unwired: 1 in]
                            n1974 = Bundle By Name("Y"=w3086, "t0"=w3085) -> (w3078:waveform(dbl))  [unwired: 1 in]
                            n1975 = Build Array(w3084, w3083, w3082, w3081, w3080, w3079, w3078) -> (w3077:waveform(dbl)[])
                            n1976 = TDMS Write(0:w3098, 5:"TEST VALUES", 7:w3069, 9:w3077) -> (4:w3068:refnum<k34>, 6:w3067:string, 15:w3066:errorcluster)  [unwired: 2 in, 1 out]
                            n1977 = TDMS Write(0:w3068, 5:w3067, 7:"TIME", 9:w3064, 11:w3066) -> (15:w3063:errorcluster)  [unwired: 1 in, 3 out]
                            n1978 = local write "data file error"(w3063) -> ()
                          }
                        }
                      }
                    }
                  }
                }
              }
              frame #2 {
                n1979 = case shown="True" w3102 {
                  tunnel: w3106 -> [_ w3111]
                  tunnel: w3105 -> [_ w3110]
                  tunnel: w3104 -> [_ w3108]
                  tunnel: w3103 -> [_ w3107]
                  frame False {
                  }
                  frame True {
                    n1980 = local read "DISP LAB02-1"() -> (w3112:T4)
                    n1981 = local read "SIG LAB02-1"() -> (w3113:T2)
                    n1982 = local read "ON L02-1"() -> (w3109:cluster{"amps":dbl, "volts":dbl, "pf":dbl})
                    n1983 = Unbundle(w3113) -> ("AMPS"=w3119:dbl, "VOLTS"=w3117:dbl, "PF"=w3116:dbl, "Tmp Live"=w3115:dbl, "Tmp Neut"=w3118:dbl)
                    n1984 = Unbundle(w3112) -> ("CYCLE"=w3114:dbl)  [unwired: 2 out]
                    n1985 = stacked-sequence {
                      tunnel: w3119 -> [w3123 w3142]
                      tunnel: w3118 -> [_ w3141]
                      tunnel: w3117 -> [w3122 w3140]
                      tunnel: w3116 -> [w3121 w3139]
                      tunnel: w3115 -> [_ w3138]
                      tunnel: w3114 -> [_ w3137]
                      tunnel: w3111 -> [_ w3136]
                      tunnel: w3110 -> [w3124 _]
                      tunnel: w3109 -> [w3120 w3134]
                      tunnel: w3108 -> [_ w3135]
                      tunnel: w3107 -> [_ w3130]
                      frame #0 {
                        n1986 = case shown="True" w3124 {
                          tunnel: w3123 -> [_ w3129]
                          tunnel: w3122 -> [_ w3128]
                          tunnel: w3121 -> [_ w3127]
                          tunnel: w3120 -> [_ w3125]
                          frame False {
                          }
                          frame True {
                            n1987 = Bundle(cluster=w3125, "amps"=w3129, "volts"=w3128, "pf"=w3127) -> (w3126:cluster{"amps":dbl, "volts":dbl, "pf":dbl})
                            n1988 = local write "ON L02-1"(w3126) -> ()
                          }
                        }
                      }
                      frame #1 {
                        n1989 = Unbundle(w3134) -> ("amps"=w3133:dbl, "volts"=w3132:dbl, "pf"=w3131:dbl)
                        n1990 = case shown="True" w3135 {
                          tunnel: w3142 -> [_ w3174]
                          tunnel: w3141 -> [_ w3181]
                          tunnel: w3140 -> [_ _]
                          tunnel: w3139 -> [_ _]
                          tunnel: w3138 -> [_ w3180]
                          tunnel: w3137 -> [_ w3179]
                          tunnel: w3136 -> [_ w3144]
                          tunnel: w3133 -> [_ w3176]
                          tunnel: w3132 -> [_ w3175]
                          tunnel: w3131 -> [_ w3173]
                          tunnel: w3130 -> [_ w3165]
                          frame False {
                          }
                          frame True {
                            n1991 = local read "TDMS LAB02-1"() -> (w3178:refnum<k34>)
                            n1992 = Build Array(w3175) -> (w3170:dbl[])
                            n1993 = Build Array(w3173) -> (w3169:dbl[])
                            n1994 = Build Array(w3180) -> (w3168:dbl[])
                            n1995 = Build Array(w3181) -> (w3167:dbl[])
                            n1996 = Build Array(w3176) -> (w3172:dbl[])
                            n1997 = Build Array(w3174) -> (w3171:dbl[])
                            n1998 = Build Array(w3179) -> (w3166:dbl[])
                            n1999 = Build Array("AMPS ON", "AMPS OFF", "VOLTS", "PF", "TEMP Live", "TEMP Neut", "CYCLE") -> (w3149:string[])
                            n2000 = Bundle By Name("Y"=w3172, "t0"=w3165) -> (w3164:waveform(dbl))  [unwired: 1 in]
                            n2001 = Bundle By Name("Y"=w3171, "t0"=w3165) -> (w3163:waveform(dbl))  [unwired: 1 in]
                            n2002 = Bundle By Name("Y"=w3170, "t0"=w3165) -> (w3162:waveform(dbl))  [unwired: 1 in]
                            n2003 = Bundle By Name("Y"=w3169, "t0"=w3165) -> (w3161:waveform(dbl))  [unwired: 1 in]
                            n2004 = Bundle By Name("Y"=w3168, "t0"=w3165) -> (w3160:waveform(dbl))  [unwired: 1 in]
                            n2005 = Bundle By Name("Y"=w3167, "t0"=w3165) -> (w3159:waveform(dbl))  [unwired: 1 in]
                            n2006 = Bundle By Name("Y"=w3166, "t0"=w3165) -> (w3158:waveform(dbl))  [unwired: 1 in]
                            n2007 = Build Array(w3164, w3163, w3162, w3161, w3160, w3159, w3158) -> (w3157:waveform(dbl)[])
                            n2008 = TDMS Write(0:w3178, 5:"TEST VALUES", 7:w3149, 9:w3157) -> (4:w3148:refnum<k34>, 6:w3147:string, 15:w3146:errorcluster)  [unwired: 2 in, 1 out]
                            n2009 = TDMS Write(0:w3148, 5:w3147, 7:"TIME", 9:w3144, 11:w3146) -> (15:w3143:errorcluster)  [unwired: 1 in, 3 out]
                            n2010 = local write "data file error"(w3143) -> ()
                          }
                        }
                      }
                    }
                  }
                }
              }
              frame #3 {
                n2011 = case shown="True" w3182 {
                  tunnel: w3186 -> [_ w3191]
                  tunnel: w3185 -> [_ w3190]
                  tunnel: w3184 -> [_ w3188]
                  tunnel: w3183 -> [_ w3187]
                  frame False {
                  }
                  frame True {
                    n2012 = local read "DISP LAB02-2"() -> (w3192:T4)
                    n2013 = local read "SIG LAB02-2"() -> (w3193:T2)
                    n2014 = local read "ON L02-2"() -> (w3189:cluster{"amps":dbl, "volts":dbl, "pf":dbl})
                    n2015 = Unbundle(w3193) -> ("AMPS"=w3199:dbl, "VOLTS"=w3197:dbl, "PF"=w3196:dbl, "Tmp Live"=w3195:dbl, "Tmp Neut"=w3198:dbl)
                    n2016 = Unbundle(w3192) -> ("CYCLE"=w3194:dbl)  [unwired: 2 out]
                    n2017 = stacked-sequence {
                      tunnel: w3199 -> [w3203 w3222]
                      tunnel: w3198 -> [_ w3221]
                      tunnel: w3197 -> [w3202 w3220]
                      tunnel: w3196 -> [w3201 w3219]
                      tunnel: w3195 -> [_ w3218]
                      tunnel: w3194 -> [_ w3217]
                      tunnel: w3191 -> [_ w3216]
                      tunnel: w3190 -> [w3204 _]
                      tunnel: w3189 -> [w3200 w3214]
                      tunnel: w3188 -> [_ w3215]
                      tunnel: w3187 -> [_ w3210]
                      frame #0 {
                        n2018 = case shown="True" w3204 {
                          tunnel: w3203 -> [_ w3209]
                          tunnel: w3202 -> [_ w3208]
                          tunnel: w3201 -> [_ w3207]
                          tunnel: w3200 -> [_ w3205]
                          frame False {
                          }
                          frame True {
                            n2019 = Bundle(cluster=w3205, "amps"=w3209, "volts"=w3208, "pf"=w3207) -> (w3206:cluster{"amps":dbl, "volts":dbl, "pf":dbl})
                            n2020 = local write "ON L02-2"(w3206) -> ()
                          }
                        }
                      }
                      frame #1 {
                        n2021 = Unbundle(w3214) -> ("amps"=w3213:dbl, "volts"=w3212:dbl, "pf"=w3211:dbl)
                        n2022 = case shown="True" w3215 {
                          tunnel: w3222 -> [_ w3254]
                          tunnel: w3221 -> [_ w3261]
                          tunnel: w3220 -> [_ _]
                          tunnel: w3219 -> [_ _]
                          tunnel: w3218 -> [_ w3260]
                          tunnel: w3217 -> [_ w3259]
                          tunnel: w3216 -> [_ w3224]
                          tunnel: w3213 -> [_ w3256]
                          tunnel: w3212 -> [_ w3255]
                          tunnel: w3211 -> [_ w3253]
                          tunnel: w3210 -> [_ w3245]
                          frame False {
                          }
                          frame True {
                            n2023 = local read "TDMS LAB02-2"() -> (w3258:refnum<k34>)
                            n2024 = Build Array(w3255) -> (w3250:dbl[])
                            n2025 = Build Array(w3253) -> (w3249:dbl[])
                            n2026 = Build Array(w3260) -> (w3248:dbl[])
                            n2027 = Build Array(w3261) -> (w3247:dbl[])
                            n2028 = Build Array(w3256) -> (w3252:dbl[])
                            n2029 = Build Array(w3254) -> (w3251:dbl[])
                            n2030 = Build Array(w3259) -> (w3246:dbl[])
                            n2031 = Build Array("AMPS ON", "AMPS OFF", "VOLTS", "PF", "TEMP Live", "TEMP Neut", "CYCLE") -> (w3229:string[])
